vi "IGC100 Bk.vi"(0 "Enable IGC100 Main":refnum<vi>, 1 "IGC100 Main Error":refnum<vi>, 2 "Communication Interval (s)":refnum<vi>, 3 "IGC100 Prep Error":refnum<vi>, 4 "QUIT":refnum<vi>, 5 "Enable IGC100 Prep":refnum<vi>, 6 "Main Status":refnum<vi>, 7 "Prep Status":refnum<vi>, 8 "IGC100 Main":refnum<visa-resource-name>="COM6", 9 "IGC100 Main Online":refnum<vi>, 10 "IGC100 Prep":refnum<visa-resource-name>="COM10", 11 "IGC100 Prep Online":refnum<vi>, 12 "Main Chamber Pressure":refnum<vi>, 13 "Log Interval (s)":refnum<vi>, 14 "Prep Chamber Pressure":refnum<vi>, 15 "Load Lock Backing Pressure":refnum<vi>) -> ()   [LabVIEW 2010]
uses:
  <vilib>/Utility/error.llb/DialogType.ctl
  <vilib>/Analysis/NI_AALBase.lvlib
panel:
  out "Error Message (Prep)":string=" INSTRUCTIONS:\r\rNormal Use:  When using subVIs that incorporate the error in/error out (or error I/O) structure, place this handler where you want to inform the user of an error, typically at the end of the I/O data path, as the last action of the program.  If the error in error? is ERROR, the handler creates a message describing the error and its source.  If the type of dialog = 1 (default), the message is displayed to the user, who can only acknowedge it.  If the type = 2, the user can acknowledge the message or abort execution; aborting a program with active I/O is not recommended.  If the type = 0, no message is displayed; this is used to process the error programmatically, and the error out cluster elements are wired to individual terminals for that reason.  \r\rOther Use:\n\r\nlocal testing.  To test the error code of a subVI or function that does not have the error I/O structure, you can wire its error code and a source string to the local error code and error source inputs.  If error in error? indicates no error and error code is not equal to 0, the local code and source are substituted for the error in values, and error? is set TRUE (ERROR)."
  out "Error Source (Prep)":string
  out "Error Code (Prep)":i32 format="%0.0f"
  out "Error Code (Main)":i32 format="%0.0f"
  out "Error Source (Main)":string
  out "Error Message (Main)":string=" INSTRUCTIONS:\r\rNormal Use:  When using subVIs that incorporate the error in/error out (or error I/O) structure, place this handler where you want to inform the user of an error, typically at the end of the I/O data path, as the last action of the program.  If the error in error? is ERROR, the handler creates a message describing the error and its source.  If the type of dialog = 1 (default), the message is displayed to the user, who can only acknowedge it.  If the type = 2, the user can acknowledge the message or abort execution; aborting a program with active I/O is not recommended.  If the type = 0, no message is displayed; this is used to process the error programmatically, and the error out cluster elements are wired to individual terminals for that reason.  \r\rOther Use:\n\r\nlocal testing.  To test the error code of a subVI or function that does not have the error I/O structure, you can wire its error code and a source string to the local error code and error source inputs.  If error in error? indicates no error and error code is not equal to 0, the local code and source are substituted for the error in values, and error? is set TRUE (ERROR)."
  # "The following errors occurred while trying to open communications."
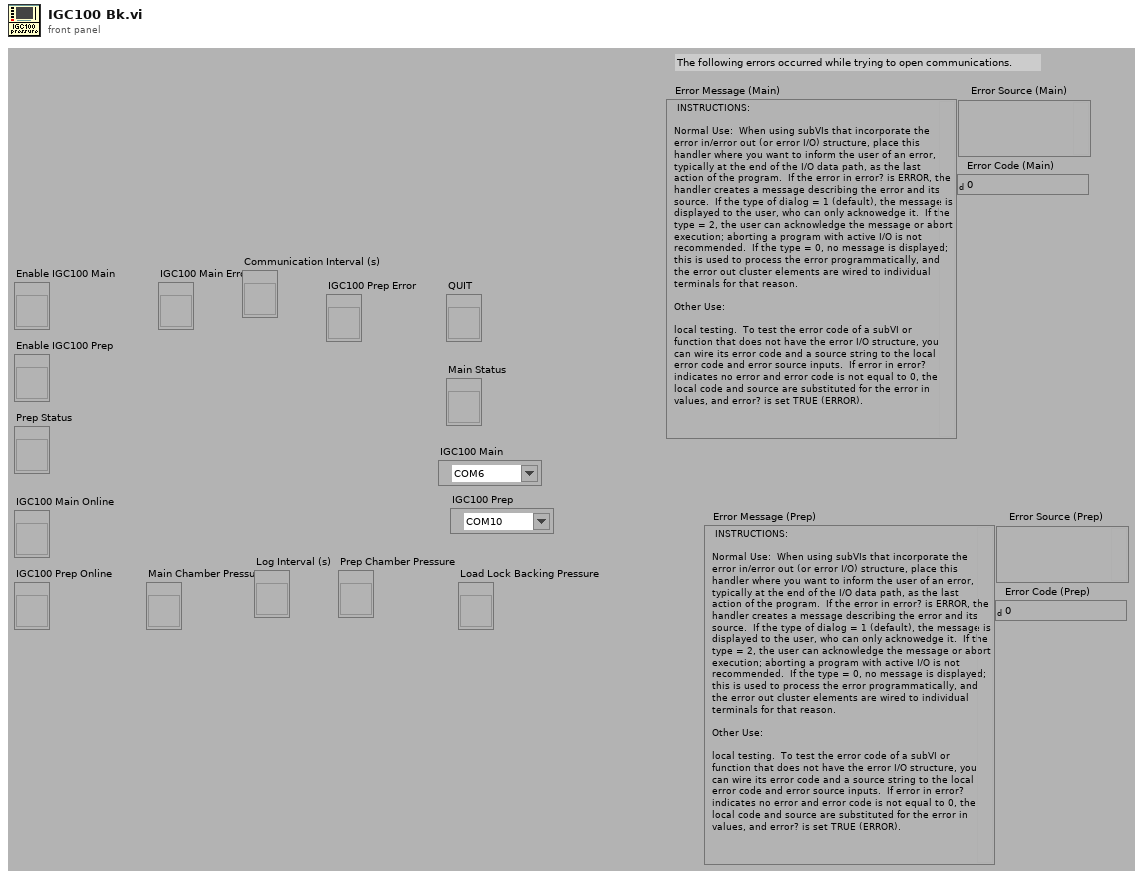
[diagram p1: front panel]
types:
  T1 = typedef "DialogType.ctl" = u16
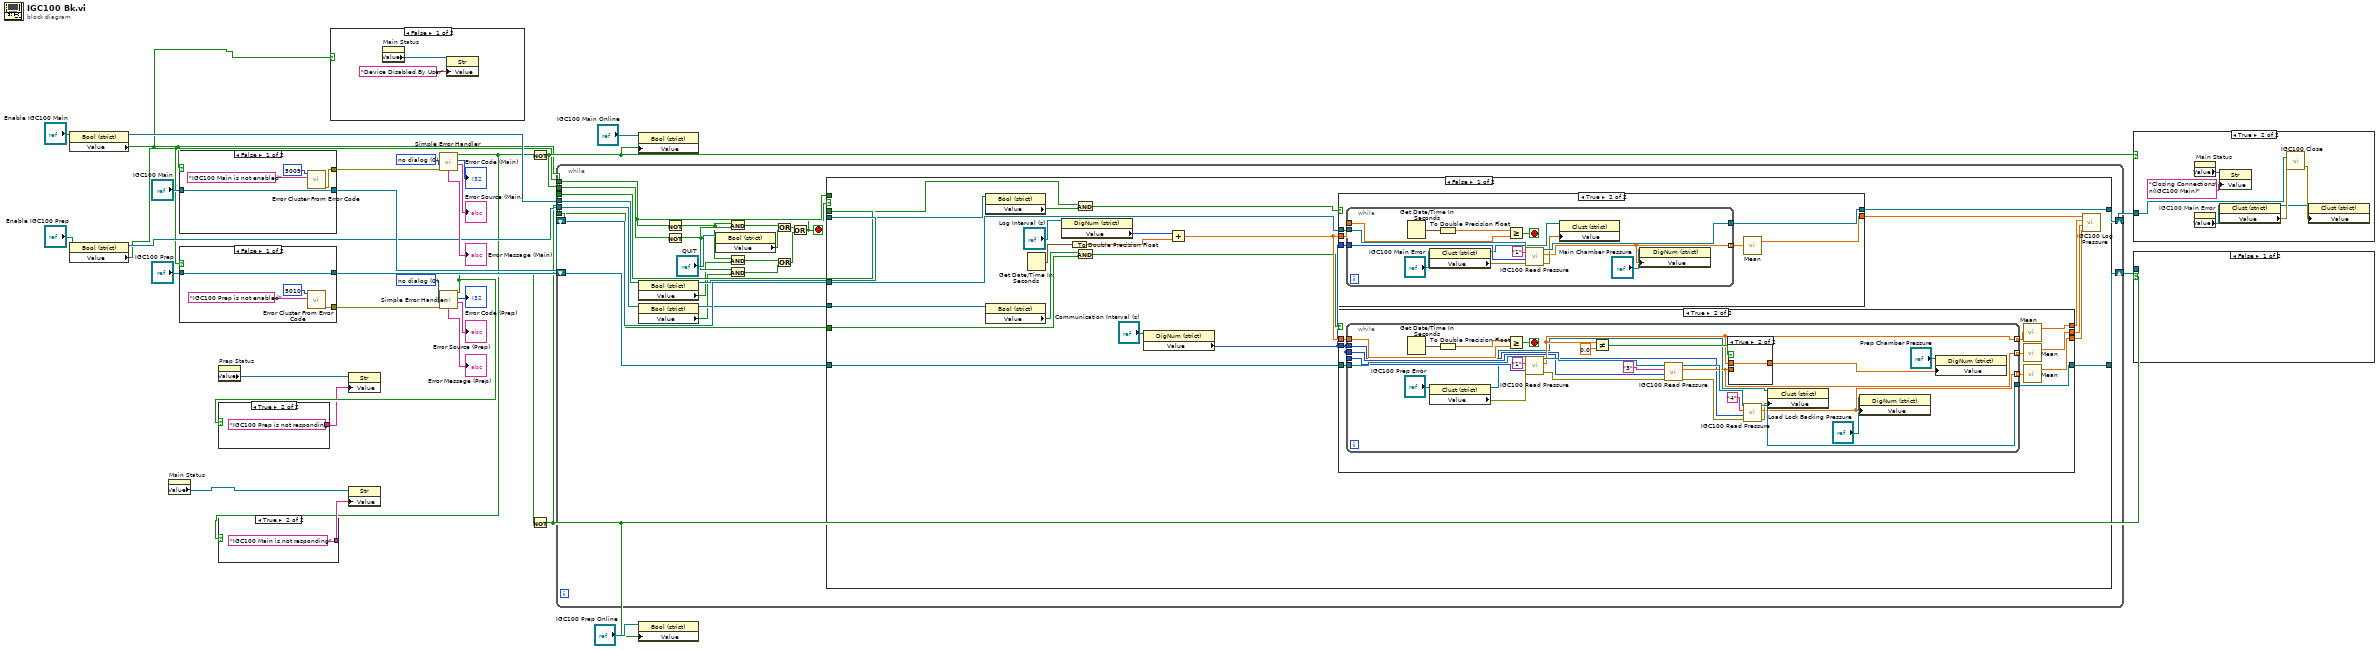
[diagram p0: block diagram]
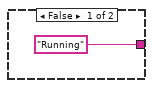
[diagram p2: hidden frame]
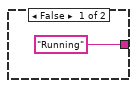
[diagram p3: hidden frame]
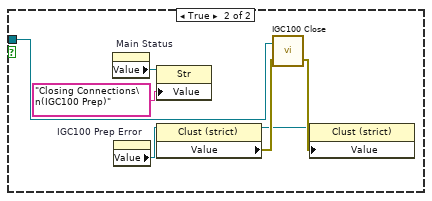
[diagram p5: hidden frame]
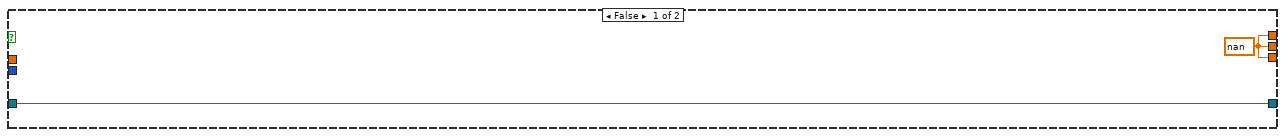
[diagram p7: hidden frame]
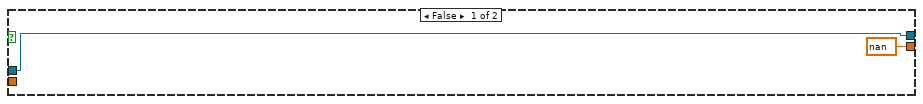
[diagram p9: hidden frame]
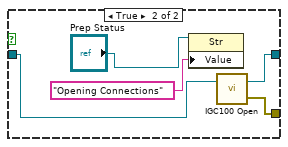
[diagram p11: hidden frame]
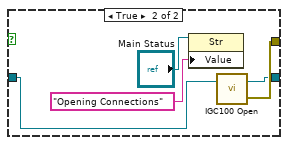
[diagram p12: hidden frame]
diagram:
  w9 = T1 0 items=["no dialog", "OK message", "continue or stop message", "OK message + warnings", "continue/stop + warnings"] ("type of dialog (OK msg:1)")
  w10 = T1 0 items=["no dialog", "OK message", "continue or stop message", "OK message + warnings", "continue/stop + warnings"] ("type of dialog (OK msg:1)")
  n1 = property on="Property Node" class="Bool (strict)"(reference="Enable IGC100 Main") -> (reference out=w16:refnum<vi>, "Value"=w1:bool)  [unwired: 1 in, 1 out]
  n2 = property on="Property Node" class="Bool (strict)"(reference="Enable IGC100 Prep") -> (reference out=w15:refnum<vi>, "Value"=w8:bool)  [unwired: 1 in, 1 out]
  n3 = property on="Main Status" class="LVObjRef (strict)"() -> ("Value"=w3:refnum<vi>)  [unwired: 2 in, 2 out]
  n4 = case shown="False" w1 {
    tunnel: "IGC100 Main" -> [w36 w41]
    tunnel: [w35 w40] -> w31
    tunnel: [w36 w39] -> w29
    frame False {
      n5 = call <vilib>:"Error Cluster From Error Code.vi"("error message (\"\")"="IGC100 Main is not enabled" ("error message (\"\")"), "error code (0)"=5009) -> ("error out"=w35:errorcluster)  [unwired: 7 in]
    }
    frame True {
      n6 = property on="Property Node" class="Str"(reference="Main Status", "Value"="Opening Connections") -> ()  [unwired: 1 in, 2 out]
      n7 = call "IGC100 Open.vi"("VISA in"=w41) -> ("error out"=w40:errorcluster, "VISA out"=w39:refnum<visa-resource-name>)  [unwired: 1 in]
    }
  }
  n8 = case shown="False" w8 {
    tunnel: "IGC100 Prep" -> [w45 w50]
    tunnel: [w42 w49] -> w19
    tunnel: [w45 w48] -> w17
    frame False {
      n9 = call <vilib>:"Error Cluster From Error Code.vi"("error message (\"\")"="IGC100 Prep is not enabled" ("error message (\"\")"), "error code (0)"=5010) -> ("error out"=w42:errorcluster)  [unwired: 7 in]
    }
    frame True {
      n10 = property on="Property Node" class="Str"(reference="Prep Status", "Value"="Opening Connections") -> ()  [unwired: 1 in, 2 out]
      n11 = call "IGC100 Open.vi"("VISA in"=w50) -> ("error out"=w49:errorcluster, "VISA out"=w48:refnum<visa-resource-name>)  [unwired: 1 in]
    }
  }
  n12 = property on="Prep Status" class="LVObjRef (strict)"() -> ("Value"=w7:refnum<vi>)  [unwired: 2 in, 2 out]
  n13 = case shown="False" w1 {
    frame False {
      n14 = property on="Main Status" class="LVObjRef (strict)"() -> ("Value"=w52:refnum<vi>)  [unwired: 2 in, 2 out]
      n15 = property on="Property Node" class="Str"(reference=w52, "Value"="Device Disabled By User") -> ()  [unwired: 1 in, 2 out]
    }
    frame True {
    }
  }
  n16 = call <vilib>:"Simple Error Handler.vi"("type of dialog (OK msg:1)"=w10, "error in (no error)"=w31) -> ("error?"=w2:bool, "code out"=→"Error Code (Main)":i32, "source out"=→"Error Source (Main)":string, "message"=→"Error Message (Main)":string)  [unwired: 3 in, 1 out]
  n17 = case shown="True" w2 {
    tunnel: ["Running" "IGC100 Main is not responding"] -> w4
    frame False {
    }
    frame True {
    }
  }
  n18 = property on="Property Node" class="Str"(reference=w3, "Value"=w4) -> ()  [unwired: 1 in, 2 out]
  n19 = call <vilib>:"Simple Error Handler.vi"("type of dialog (OK msg:1)"=w9, "error in (no error)"=w19) -> ("error?"=w6:bool, "code out"=→"Error Code (Prep)":i32, "source out"=→"Error Source (Prep)":string, "message"=→"Error Message (Prep)":string)  [unwired: 3 in, 1 out]
  n20 = case shown="True" w6 {
    tunnel: ["Running" "IGC100 Prep is not responding"] -> w5
    frame False {
    }
    frame True {
    }
  }
  n21 = property on="Property Node" class="Str"(reference=w7, "Value"=w5) -> ()  [unwired: 1 in, 2 out]
  n22 = Not(x=w2) -> (.not. x?=w12:bool)
  n23 = Not(x=w6) -> (.not. x?=w11:bool)
  n24 = while {
    shift-right: [w78] -> w13
    shift-left: w29 -> [w77]
    shift-right: [w79] -> w14
    shift-left: w17 -> [w80]
    tunnel: w1 -> [w67]
    tunnel: w16 -> [w75]
    tunnel: w15 -> [w74]
    tunnel: w12 -> [w69]
    tunnel: w11 -> [w68]
    tunnel: w8 -> [w66]
    stop <- w57 stop-if-true
    n25 = property on="Property Node" class="Bool (strict)"(reference=w75) -> (reference out=w71:refnum<vi>, "Value"=w62:bool)  [unwired: 1 in, 1 out]
    n26 = property on="Property Node" class="Bool (strict)"(reference=w74) -> (reference out=w70:refnum<vi>, "Value"=w64:bool)  [unwired: 1 in, 1 out]
    n27 = Not(x=w67) -> (.not. x?=w63:bool)
    n28 = Not(x=w66) -> (.not. x?=w65:bool)
    n29 = property on="Property Node" class="Bool (strict)"(reference="QUIT") -> ("Value"=w72:bool)  [unwired: 1 in, 2 out]
    n30 = And(x=w63, y=w65) -> (x .and. y?=w73:bool)
    n31 = And(x=w63, y=w62) -> (x .and. y?=w60:bool)
    n32 = And(x=w65, y=w64) -> (x .and. y?=w61:bool)
    n33 = Or(x=w73, y=w72) -> (x .or. y?=w58:bool)
    n34 = Or(x=w60, y=w61) -> (x .or. y?=w59:bool)
    n35 = Or(x=w58, y=w59) -> (x .or. y?=w57:bool)
    n36 = case shown="False" w57 {
      tunnel: w80 -> [w103 w169]
      tunnel: [w102 w169] -> w79
      tunnel: w77 -> [w101 w168]
      tunnel: [w100 w168] -> w78
      tunnel: w67 -> [_ _]
      tunnel: w71 -> [w92 _]
      tunnel: w70 -> [w91 _]
      tunnel: w69 -> [w81 _]
      tunnel: w68 -> [w82 _]
      frame False {
        n37 = property on="Property Node" class="Bool (strict)"(reference=w92) -> ("Value"=w83:bool)  [unwired: 1 in, 2 out]
        n38 = property on="Property Node" class="Bool (strict)"(reference=w91) -> ("Value"=w84:bool)  [unwired: 1 in, 2 out]
        n39 = Get Date/Time In Seconds() -> (seconds since 1Jan1904=w95:timestamp)
        n40 = property on="Property Node" class="DigNum (strict)"(reference="Log Interval (s)") -> ("Value"=w88:u32)  [unwired: 1 in, 2 out]
        n41 = To Double Precision Float(number=w95) -> (double precision float=w94:dbl)
        n42 = And(x=w81, y=w83) -> (x .and. y?=w89:bool)
        n43 = And(x=w84, y=w82) -> (x .and. y?=w90:bool)
        n44 = property on="Property Node" class="DigNum (strict)"(reference="Communication Interval (s)") -> ("Value"=w86:u32)  [unwired: 1 in, 2 out]
        n45 = Add(x=w88, y=w94) -> (x+y=w93:dbl)
        n46 = case shown="True" w89 {
          tunnel: w101 -> [w147 w153]
          tunnel: [w147 w152] -> w100
          tunnel: [nan ("mean") w150] -> w99
          tunnel: w93 -> [_ w149]
          tunnel: w86 -> [_ w148]
          frame False {
          }
          frame True {
            n47 = while {
              tunnel: w153 -> [w166]
              tunnel: [w165] -> w152
              tunnel: [w156] -> w151 mode=indexing
              tunnel: w149 -> [w161]
              tunnel: w148 -> [w160]
              stop <- w163 stop-if-true
              n48 = Get Date/Time In Seconds() -> (seconds since 1Jan1904=w162:timestamp)
              n49 = property on="Property Node" class="Clust (strict)"(reference="IGC100 Main Error") -> (reference out=w157:refnum<vi>, "Value"=w159:errorcluster)  [unwired: 1 in, 1 out]
              n50 = To Double Precision Float(number=w162) -> (double precision float=w164:dbl)
              n51 = Greater Or Equal?(x=w164, y=w161) -> (x >= y?=w163:bool)
              n52 = call "IGC100 Read Pressure.vi"("error in"=w159, "Communication Interval (ms)"=w160, "Channel"="1", "VISA in"=w166) -> ("error out"=w158:errorcluster, "Pressure"=w156:dbl, "VISA out"=w165:refnum<visa-resource-name>)  [unwired: 1 in]
              n53 = property on="Property Node" class="Clust (strict)"(reference=w157, "Value"=w158) -> ()  [unwired: 1 in, 2 out]
              n54 = property on="Property Node" class="DigNum (strict)"(reference="Main Chamber Pressure", "Value"=w156) -> ()  [unwired: 1 in, 2 out]
            }
            n55 = call <vilib>:"Mean.vi"("X"=w151) -> ("mean"=w150:dbl)  [unwired: 1 out]
          }
        }
        n56 = case shown="True" w90 {
          tunnel: w103 -> [w105 w115]
          tunnel: [w105 w114] -> w102
          tunnel: [w104 w110] -> w98
          tunnel: [w104 w109] -> w97
          tunnel: [w104 w108] -> w96
          tunnel: w93 -> [_ w107]
          tunnel: w86 -> [_ w106]
          frame False {
            w104 = nan ("mean")
          }
          frame True {
            n57 = while {
              tunnel: w115 -> [w143]
              tunnel: [w142] -> w114
              tunnel: [w134] -> w111 mode=indexing
              tunnel: [w133] -> w112 mode=indexing
              tunnel: [w117] -> w113 mode=indexing
              tunnel: w107 -> [w129]
              tunnel: w106 -> [w126]
              tunnel: w106 -> [w125]
              tunnel: w106 -> [w124]
              stop <- w131 stop-if-true
              n58 = Get Date/Time In Seconds() -> (seconds since 1Jan1904=w130:timestamp)
              n59 = property on="Property Node" class="Clust (strict)"(reference="IGC100 Prep Error") -> (reference out=w120:refnum<vi>, "Value"=w123:errorcluster)  [unwired: 1 in, 1 out]
              n60 = To Double Precision Float(number=w130) -> (double precision float=w132:dbl)
              n61 = Greater Or Equal?(x=w132, y=w129) -> (x >= y?=w131:bool)
              n62 = call "IGC100 Read Pressure.vi"("error in"=w123, "Communication Interval (ms)"=w126, "Channel"="1", "VISA in"=w143) -> ("error out"=w128:errorcluster, "Pressure"=w134:dbl, "VISA out"=w140:refnum<visa-resource-name>)  [unwired: 1 in]
              n63 = Not Equal?(x=w134, y=0.0) -> (x != y?=w136:bool)
              n64 = call "IGC100 Read Pressure.vi"("error in"=w128, "Communication Interval (ms)"=w125, "Channel"="3", "VISA in"=w140) -> ("error out"=w127:errorcluster, "Pressure"=w133:dbl, "VISA out"=w141:refnum<visa-resource-name>)  [unwired: 1 in]
              n65 = case shown="True" w136 {
                tunnel: w134 -> [_ w145]
                tunnel: [w144 w145] -> w119
                tunnel: w133 -> [w144 _]
                frame False {
                }
                frame True {
                }
              }
              n66 = call "IGC100 Read Pressure.vi"("error in"=w127, "Communication Interval (ms)"=w124, "Channel"="4", "VISA in"=w141) -> ("error out"=w122:errorcluster, "Pressure"=w117:dbl, "VISA out"=w142:refnum<visa-resource-name>)  [unwired: 1 in]
              n67 = property on="Property Node" class="Clust (strict)"(reference=w120, "Value"=w122) -> ()  [unwired: 1 in, 2 out]
              n68 = property on="Property Node" class="DigNum (strict)"(reference="Load Lock Backing Pressure", "Value"=w117) -> ()  [unwired: 1 in, 2 out]
              n69 = property on="Property Node" class="DigNum (strict)"(reference="Prep Chamber Pressure", "Value"=w119) -> ()  [unwired: 1 in, 2 out]
            }
            n70 = call <vilib>:"Mean.vi"("X"=w111) -> ("mean"=w110:dbl)  [unwired: 1 out]
            n71 = call <vilib>:"Mean.vi"("X"=w112) -> ("mean"=w109:dbl)  [unwired: 1 out]
            n72 = call <vilib>:"Mean.vi"("X"=w113) -> ("mean"=w108:dbl)  [unwired: 1 out]
          }
        }
        n73 = call "IGC100 Log Pressure.vi"("Load Lock Backing Pressure (Convectron)"=w96, "Prep Pressure (Convectron)"=w97, "Prep Pressure (Ion)"=w98, "Main Pressure (Ion)"=w99) -> ()  [unwired: 8 in]
      }
      frame True {
      }
    }
  }
  n74 = property on="Property Node" class="Bool (strict)"(reference="IGC100 Main Online", "Value"=w12) -> ()  [unwired: 1 in, 2 out]
  n75 = property on="Property Node" class="Bool (strict)"(reference="IGC100 Prep Online", "Value"=w11) -> ()  [unwired: 1 in, 2 out]
  n76 = case shown="True" w12 {
    tunnel: w13 -> [_ w176]
    frame False {
    }
    frame True {
      n77 = property on="Main Status" class="LVObjRef (strict)"() -> ("Value"=w171:refnum<vi>)  [unwired: 2 in, 2 out]
      n78 = property on="IGC100 Main Error" class="LVObjRef (strict)"() -> ("Value"=w172:refnum<vi>)  [unwired: 2 in, 2 out]
      n79 = property on="Property Node" class="Str"(reference=w171, "Value"="Closing Connections\n(IGC100 Main)") -> ()  [unwired: 1 in, 2 out]
      n80 = property on="Property Node" class="Clust (strict)"(reference=w172) -> (reference out=w173:refnum<vi>, "Value"=w174:errorcluster)  [unwired: 1 in, 1 out]
      n81 = call "IGC100 Close.vi"("error in"=w174, "VISA in"=w176) -> ("error out"=w175:errorcluster)  [unwired: 1 in]
      n82 = property on="Property Node" class="Clust (strict)"(reference=w173, "Value"=w175) -> ()  [unwired: 1 in, 2 out]
    }
  }
  n83 = case shown="False" w11 {
    tunnel: w14 -> [_ w183]
    frame False {
    }
    frame True {
      n84 = property on="Main Status" class="LVObjRef (strict)"() -> ("Value"=w178:refnum<vi>)  [unwired: 2 in, 2 out]
      n85 = property on="IGC100 Prep Error" class="LVObjRef (strict)"() -> ("Value"=w179:refnum<vi>)  [unwired: 2 in, 2 out]
      n86 = property on="Property Node" class="Str"(reference=w178, "Value"="Closing Connections\n(IGC100 Prep)") -> ()  [unwired: 1 in, 2 out]
      n87 = property on="Property Node" class="Clust (strict)"(reference=w179) -> (reference out=w180:refnum<vi>, "Value"=w181:errorcluster)  [unwired: 1 in, 1 out]
      n88 = call "IGC100 Close.vi"("error in"=w181, "VISA in"=w183) -> ("error out"=w182:errorcluster)  [unwired: 1 in]
      n89 = property on="Property Node" class="Clust (strict)"(reference=w180, "Value"=w182) -> ()  [unwired: 1 in, 2 out]
    }
  }
